vi "lookup_coordinates.vi"(8 "error in (no error)":errorcluster, 9 "frame index":i32, 10 "position coordinates":dbl[][](array[numeric]), 11 "PositionSignals in":refnum<class "PositionSignals.lvclass">) -> (0 "error out":errorcluster, 2 "pixel coordinates":i32[][](array[numeric]), 3 "PositionSignals out":refnum<class "PositionSignals.lvclass">)   [LabVIEW 2010, in "PositionSignals.lvclass"]
uses:
  PositionSignals.lvclass
  common/classes/Image/Image/pixel_position_cluster.ctl
  common/classes/Image/Image/Image.lvclass
  common/classes/Image/Image/pixel_positions_cluster.ctl
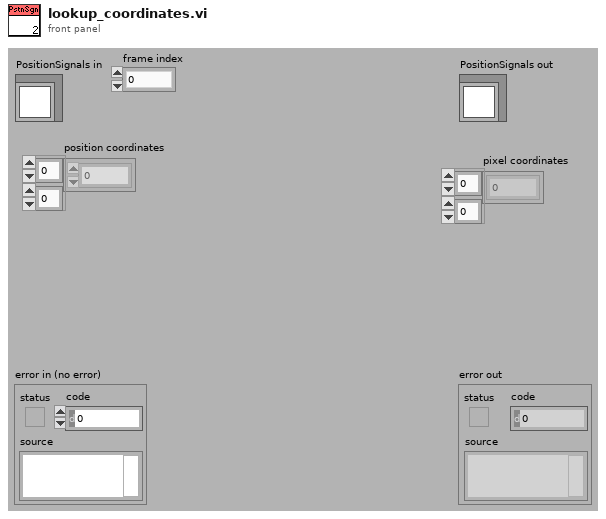
[diagram p1: front panel]
types:
  T1 = typedef "Image.lvclass/pixel_position_cluster.ctl" = cluster{"x":dbl, "y":dbl}
  T2 = typedef "Image.lvclass/pixel_positions_cluster.ctl" = cluster{"x":dbl[], "y":dbl[], "z":dbl}
  T3 = cluster{"Line End Points":cluster{"X":dbl, "Y":dbl}[]}
  T4 = cluster{"Line End Points":cluster{"X":dbl, "Y":dbl}[]}[]
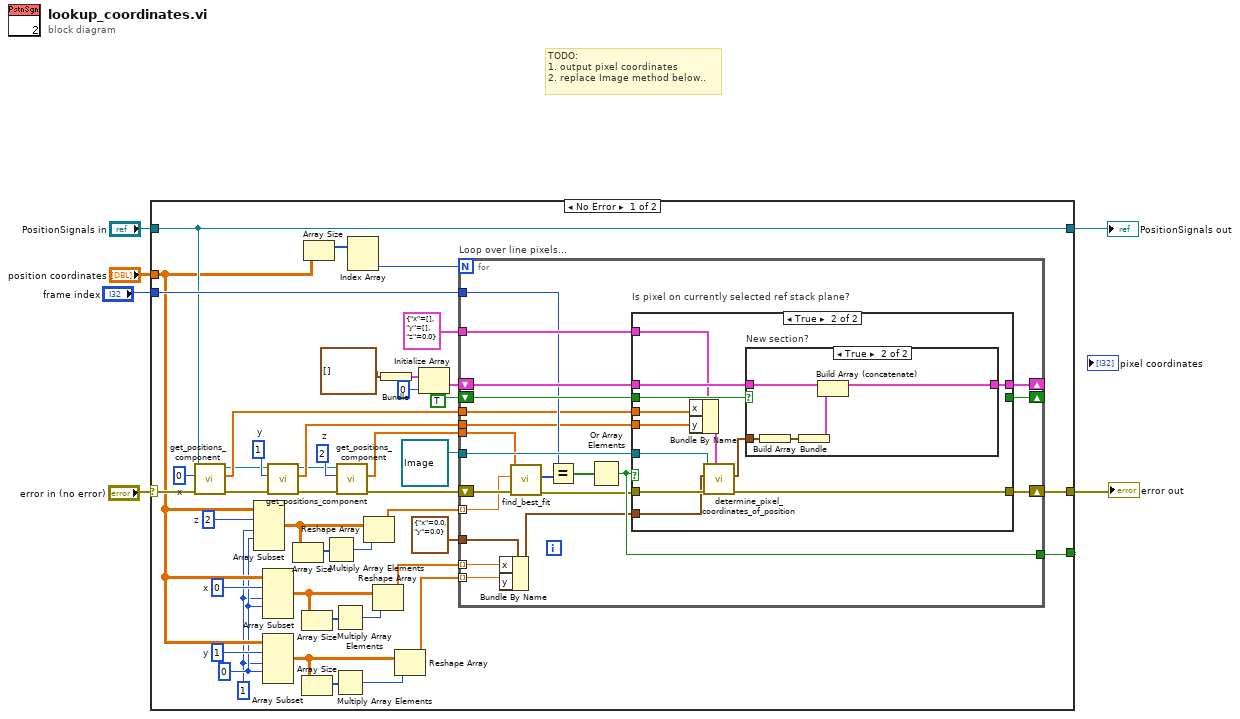
[diagram p0: block diagram]
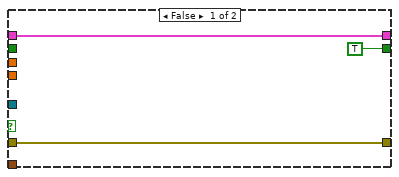
[diagram p2: hidden frame]
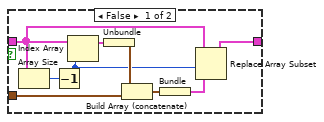
[diagram p3: hidden frame]
diagram:
  # "TODO:\n1. output pixel coordinates\n2. replace Image method below.."
  n1 = case shown="No Error" "error in (no error)" {
    selector: "error in (no error)" -> [w26 w102]
    tunnel: "frame index" -> [w44 _]
    tunnel: [w40 w102] -> w4
    tunnel: [w50 _] -> _
    tunnel: "PositionSignals in" -> [w29 w101]
    tunnel: [w29 w101] -> w1
    tunnel: "position coordinates" -> [w11 _]
    frame No Error {
      w12 = 1  # y
      w7 = 1 ("length")
      w19 = 0  # x
      w8 = 0 ("index")
      w21 = 2  # z
      w33 = 0  # x
      w34 = 1  # y
      w36 = 2  # z
      n2 = call "get_positions_component.vi"("error in (no error)"=w26, "dimension (0/1/2 for x/y/z)"=w33, "PositionSignals in"=w29) -> ("error out"=w27:errorcluster, "x positions"=w32:sgl[], "PositionSignals out"=w28:refnum<class "PositionSignals.lvclass">)  [unwired: 6 in]
      n3 = Array Subset(array=w11, index (row)=w21, length (row)=w7, index (col)=w8) -> (w24:dbl[][])  [unwired: 1 in]
      n4 = Array Subset(array=w11, index (row)=w19, length (row)=w7, index (col)=w8) -> (w16:dbl[][])  [unwired: 1 in]
      n5 = Array Subset(array=w11, index (row)=w12, length (row)=w7, index (col)=w8) -> (w15:dbl[][])  [unwired: 1 in]
      n6 = call "get_positions_component.vi"("error in (no error)"=w27, "dimension (0/1/2 for x/y/z)"=w34, "PositionSignals in"=w28) -> ("error out"=w25:errorcluster, "x positions"=w31:sgl[], "PositionSignals out"=w30:refnum<class "PositionSignals.lvclass">)  [unwired: 6 in]
      n7 = Array Size(array=w24) -> (size(s)=w22:i32[])
      n8 = Array Size(array=w16) -> (size(s)=w18:i32[])
      n9 = Array Size(array=w15) -> (size(s)=w13:i32[])
      n10 = Array Size(array=w11) -> (size(s)=w39:i32[])
      n11 = Multiply Array Elements(1:w22) -> (0:w23:i32)
      n12 = Multiply Array Elements(1:w18) -> (0:w17:i32)
      n13 = Multiply Array Elements(1:w13) -> (0:w14:i32)
      n14 = call "get_positions_component.vi"("error in (no error)"=w25, "dimension (0/1/2 for x/y/z)"=w36, "PositionSignals in"=w30) -> ("error out"=w37:errorcluster, "x positions"=w35:sgl[])  [unwired: 6 in, 1 out]
      n15 = Index Array(array=w39) -> (element #2=w38:i32)  [unwired: 2 in, 1 out]
      n16 = Reshape Array(w24, w23) -> (w20:dbl[])
      n17 = Reshape Array(w16, w17) -> (w10:dbl[])
      n18 = Bundle("Line End Points"=cluster{"X":dbl, "Y":dbl}[] []) -> (w42:T3)  [unwired: 1 in]
      n19 = Reshape Array(w15, w14) -> (w9:dbl[])
      n20 = Initialize Array(w42, 0 ("dimension size")) -> (w41:T4)
      n21 = for "Loop over line pixels..." {
        N: w38 -> [_]
        shift-right: [w71] -> w40
        shift-left: w37 -> [w64]
        shift-right: [w69] -> _
        shift-left: w41 -> [w70]
        tunnel: w44 -> [w61]
        tunnel: w35 -> [w63]
        tunnel: [w60] -> w50
        tunnel: w20 -> [w55] mode=indexing
        shift-right: [w67] -> _
        shift-left: TRUE -> [w68]
        tunnel: T2 {"x"=[], "y"=[], "z"=0.0} ("pixel positions") -> [w66]
        tunnel: refnum<class "Image.lvclass"> refnum ("Image.lvclass") -> [w65]
        tunnel: T1 {"x"=0.0, "y"=0.0} ("pixel position") -> [w52]
        tunnel: w32 -> [w57]
        tunnel: w31 -> [w56]
        tunnel: w10 -> [w54] mode=indexing
        tunnel: w9 -> [w53] mode=indexing
        n22 = Bundle By Name(cluster=w52, "x"=w54, "y"=w53) -> (w51:T1)
        n23 = call "find_best_fit.vi"("error in (no error)"=w64, "value to be found"=w55, "search space"=w63) -> ("error out"=w58:errorcluster, "indices of fits"=w62:i32[])  [unwired: 6 in, 1 out]
        n24 = Equal?(x=w61, y=w62) -> (x = y?=w59:bool[])
        n25 = Or Array Elements(Boolean array=w59) -> (logical OR=w60:bool)
        n26 = case "Is pixel on currently selected ref stack plane?" shown="True" w60 {
          tunnel: w58 -> [w74 w86]
          tunnel: [w74 w85] -> w71
          tunnel: w70 -> [w73 w83]
          tunnel: [w73 w84] -> w69
          tunnel: w68 -> [_ w81]
          tunnel: [TRUE _] -> w67
          tunnel: w66 -> [_ w80]
          tunnel: w65 -> [_ w79]
          tunnel: w57 -> [_ w77]
          tunnel: w56 -> [_ w76]
          tunnel: w51 -> [_ w75]
          frame False {
          }
          frame True {
            n27 = Bundle By Name(cluster=w80, "x"=w77, "y"=w76) -> (w78:T2)
            n28 = call "determine_pixel_coordinates_of_position.vi"("pixel positions"=w78, "error in (no error)"=w86, "pixel position"=w75, "Image in"=w79) -> ("error out"=w85:errorcluster, "Point Coordinates"=w82:cluster{"X":dbl, "Y":dbl})  [unwired: 5 in, 1 out]
            n29 = case "New section?" shown="True" w81 {
              tunnel: [w87 w100] -> w84
              tunnel: w83 -> [w90 w99]
              tunnel: w82 -> [w93 w98]
              frame False {
                n30 = Array Size(array=w90) -> (size(s)=w95:i32)
                n31 = Decrement(x=w95) -> (x-1=w88:i32)
                n32 = Index Array(array=w90, index=w88) -> (element=w94:T3)
                n33 = Unbundle(w94) -> ("Line End Points"=w92:cluster{"X":dbl, "Y":dbl}[])
                n34 = Build Array (concatenate)(w92, w93) -> (w91:cluster{"X":dbl, "Y":dbl}[])
                n35 = Bundle(w91) -> (w89:cluster{cluster{"X":dbl, "Y":dbl}[]})  [unwired: 1 in]
                n36 = Replace Array Subset(array=w90, new element=w89, index=w88) -> (w87:T4)
              }
              frame True {
                n37 = Build Array(w98) -> (w97:cluster{"X":dbl, "Y":dbl}[])
                n38 = Bundle(w97) -> (w96:cluster{cluster{"X":dbl, "Y":dbl}[]})  [unwired: 1 in]
                n39 = Build Array (concatenate)(w99, w96) -> (w100:T4)
              }
            }
          }
        }
      }
    }
    frame Error {
    }
  }
  "error out" <- w4
  "PositionSignals out" <- w1
